vi "Auto Set Arm Angle.vi"(8 "error in":errorcluster, 10 "Arm State":T2=enum."Level", 11 "Auto Notifiers In":T1) -> (0 "error out":errorcluster, 3 "Auto Notifiers Out":T1)   [LabVIEW 2014]
doc: "Sets the Arm Angle from a Typedef"
uses:
  Main/Arms/Arm State.ctl
  Auto Notifiers.ctl
  Main/Arms/Arm clapper state.ctl
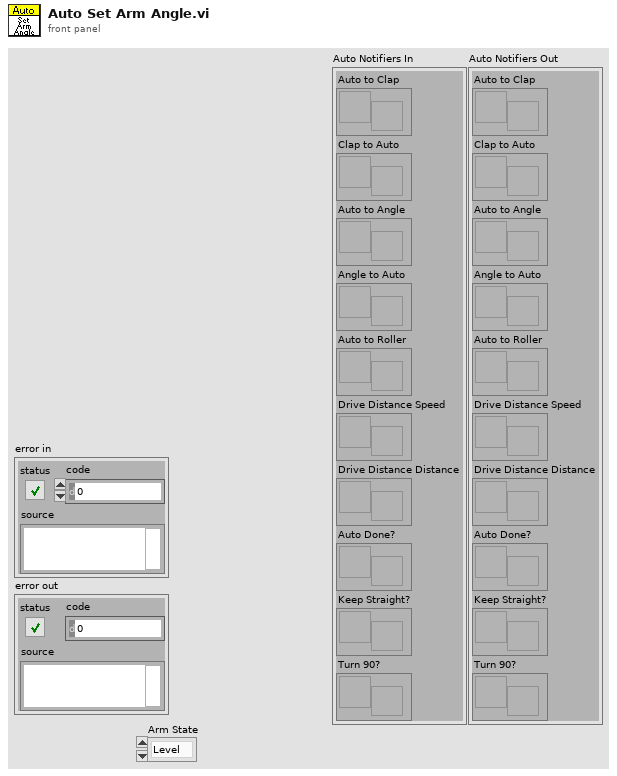
[diagram p1: front panel]
types:
  T1 = typedef "Auto Notifiers.ctl" = cluster{"Auto to Clap":refnum<notifier>, "Clap to Auto":refnum<notifier>, "Auto to Angle":refnum<notifier>, "Angle to Auto":refnum<notifier>, "Auto to Roller":refnum<notifier>, "Drive Distance Speed":refnum<notifier>, "Drive Distance Distance":refnum<notifier>, "Auto Done?":refnum<notifier>, "Keep Straight?":refnum<notifier>, "Turn 90?":refnum<notifier>}
  T2 = typedef "Arm State.ctl" = enum16{"Ground", "Level", "Feeder", "Vertical"}
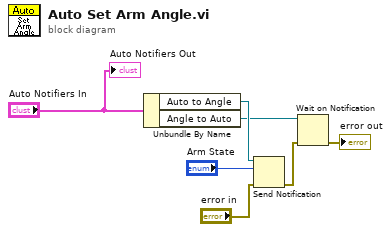
[diagram p0: block diagram]
diagram:
  n1 = Unbundle By Name("Auto Notifiers In") -> ("Auto to Angle"=w2:refnum<notifier>, "Angle to Auto"=w1:refnum<notifier>)
  n2 = Send Notification(notification="Arm State", notifier=w2, error in (no error)="error in") -> (error out=w3:errorcluster)  [unwired: 1 out]
  n3 = Wait on Notification(notifier=w1, error in (no error)=w3) -> (error out=→"error out":errorcluster)  [unwired: 2 in, 3 out]
  "Auto Notifiers Out" <- "Auto Notifiers In"
